vi "MainGUI.vi"() -> ()   [LabVIEW 2018]
uses:
  General/Controls/Queue Manager Actions.ctl
  General/Controls/MessagePacket.ctl
  General/Controls/QueueNames.ctl
  General/Controls/FGV Actions.ctl
  Hardware Mfg/Main Scan Processor Status.vi
  General/Controls/ScanType.ctl
  General/Controls/Set Get Controls.ctl
  Hardware Mfg/Thorlabs Translation Stages/Controls/Motion Translation Module Control.ctl
  Hardware Mfg/Axsun Laser/Axsun action.ctl
  Hardware Mfg/AlazarTech SDK/Controls/Alazar Engine Actions.ctl
  General/Controls/Optical Parameters.ctl
  General/Controls/Vibratome Parameters.ctl
  General/Controls/Scan Direction.ctl
  General/Controls/Imaging Parameters.ctl
panel:
  in  "Status":string
  in  "Quit":bool
  in  "Scan Type":T1
  in  "Acquire":bool
  in  "Control Panel":enum32{"Scan", "Config", "Manual Contorls"}(tab)
  in  "Imaging Parameter":T2={"Raster Scan Direction"=enum."Bi Directional", "Pixel Dwell Time [Clock Cycles]"=1, "Flyback Time [Clock Cycles]"=0, "XY Center [um]"={"X"=1.0, "Y"=1.0}, "Pixel Step Size [um]"=1.0, "XY Image Size"=enum."256 x 256", "Custom"=FALSE, "Custom Size"={"X"=1, "Y"=1}, "Line Averages"=1} {"Line Averages" min=1 max=30 step=1; "Flyback Time [Clock Cycles]" max=10 step=1; "Pixel Step Size [um]" min=0.0 max=10.0 step=0.01; "Custom Size"."Y" min=1 max=30 step=1; "Custom Size"."X" min=1 max=30 step=1; "XY Center [um]"."Y" min=1.0 max=30.0 step=1.0; "XY Center [um]"."X" min=1.0 max=30.0 step=1.0; "Pixel Dwell Time [Clock Cycles]" max=10 step=1}
  in  "Vibratome":T4={"Z Bottom [mm]"=0.0, "Pre Cut Dwell [s]"=0.0, "Blade Frequency [RPM]"=0, "Slice Speed [mm/s]"=0.0, "Post Cut Dwell [s]"=0.0, "Ramp Time [s]"=0.0, "Start X [mm]"=0.0, "Start Y [mm]"=0.0, "Slice Length [mm]"=0.0, "Slice Axis"=enum."X Axis", "Controller VISA Ref"="COM4"}
  in  "Optical Parameters":T5
  in  "Center Galvos":bool
  out "Label Name":string[][](array[string])
  out "Control Class ID":u32[](array[numeric])
  out "Image":T6(plugin-control)
  # "Image Settings"
  # "X"
  # "X"
  # "Vibratome Settings"
  # "Optical Settings"
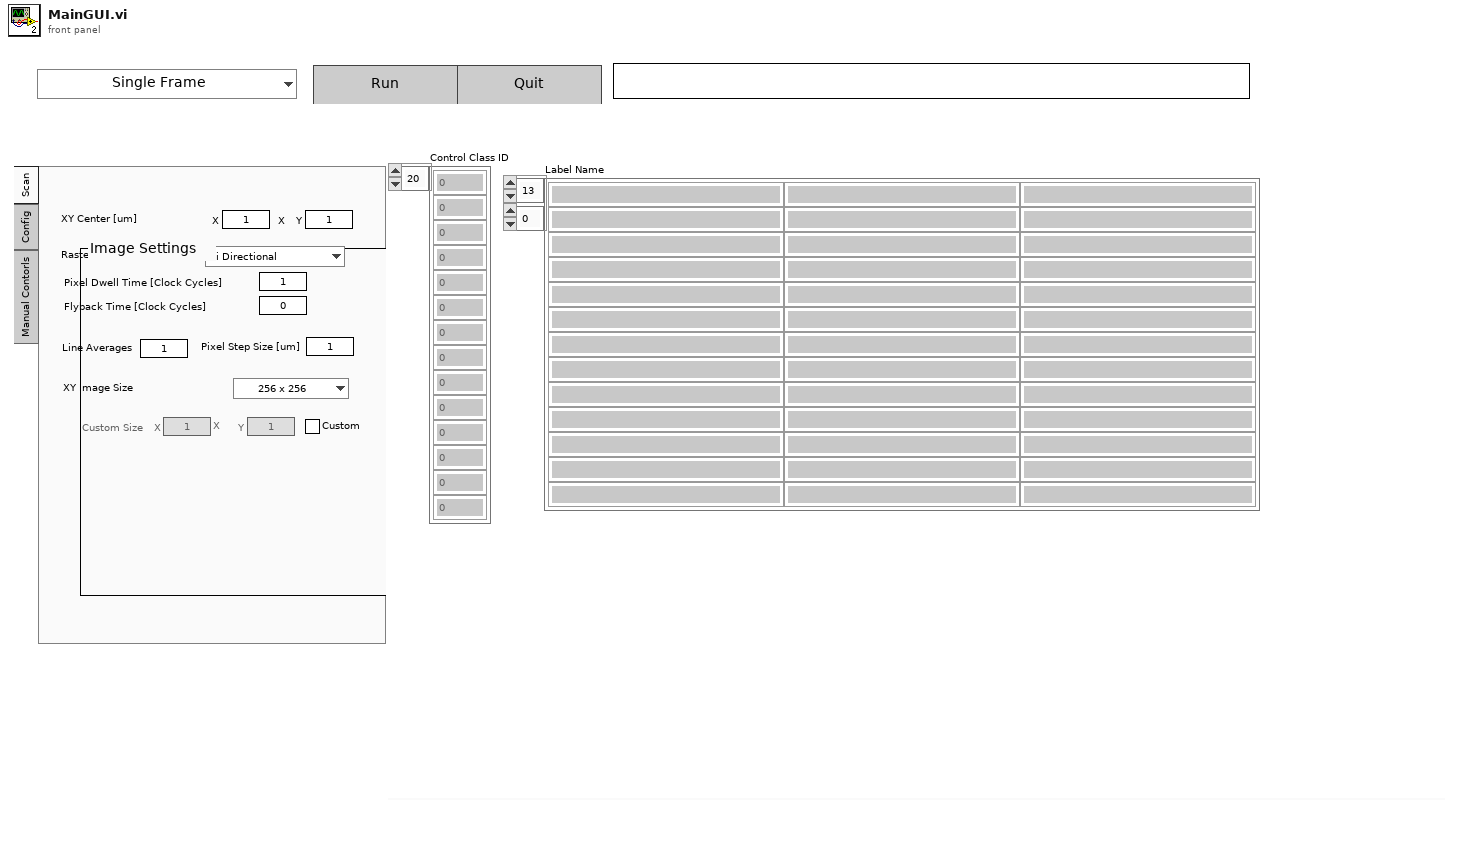
[diagram p1: front panel]
types:
  T1 = typedef "ScanType.ctl" = enum16{"Single Frame", "Continuous Frame", "ROI Line", "Vibratome", "Mosaic", "Mosaic + Slice"}
  T2 = typedef "Imaging Parameters.ctl" = cluster{"Raster Scan Direction":T3, "Pixel Dwell Time [Clock Cycles]":u16, "Flyback Time [Clock Cycles]":u16, "XY Center [um]":cluster{"X":dbl, "Y":dbl}, "Pixel Step Size [um]":dbl, "XY Image Size":enum16{"32 x 32", "64 x 64", "128 x 128", "256 x 256", "512 x 512", "1024 x 1024", "2048 x 2048"}, "Custom":bool, "Custom Size":cluster{"X":u16, "Y":u16}, "Line Averages":u8}
  T3 = typedef "Scan Direction.ctl" = enum16{"Uni Directional", "Bi Directional", "None"}
  T4 = typedef "Vibratome Parameters.ctl" = cluster{"Z Bottom [mm]":dbl, "Pre Cut Dwell [s]":dbl, "Blade Frequency [RPM]":u16, "Slice Speed [mm/s]":dbl, "Post Cut Dwell [s]":dbl, "Ramp Time [s]":dbl, "Start X [mm]":dbl, "Start Y [mm]":dbl, "Slice Length [mm]":dbl, "Slice Axis":enum16{"X Axis", "Y Axis", "Z Axis"}, "Controller VISA Ref":refnum<visa-resource-name>}
  T5 = typedef "Optical Parameters.ctl" = cluster{"Obj. Focal Length [mm]":dbl, "Scan Lens EFL[mm]":dbl, "Tube Lens EFL[mm]":dbl, "Galvo V Range (+/-)":dbl, "Galvo Max Half Angle [Deg]":dbl, "Max Galvo Range[%]":dbl}
  T6 = typedef "IMAQ Image.ctl" = refnum<image>
  T7 = typedef "QueueNames.ctl" = enum16{"Main GUI", "Main Scan Processor", "Main Display", "Main Table Stage GUI", "Main Table Stage Proc.", "Scan Engine", "Vibratome GUI", "Vibratome Processor", "Slice Engine"}
  T8 = typedef "Queue Manager Actions.ctl" = enum16{"Init", "Enqueue", "Enqueue All", "Preview Queue", "Dequeue", "Get Status", "Flush Queue", "Flush All Queues", "Release All Queues", "Release Queue", "Enqueue at Opposite End"}
  T9 = typedef "MessagePacket.ctl" = cluster{"Message":string, "Parameter":variant}
  T10 = typedef "FGV Actions.ctl" = enum16{"Init", "Set", "Get", "Clear"}
  T11 = typedef "System Parameters.ctl" = cluster{"Optical Parameters":T5, "Vibratome":T4, "Table Stages":T12, "Imaging Parameter":T2}
  T12 = typedef "Translation Stage Parameters.ctl" = cluster{"X Stage":T13, "Y Stage":T13, "Z Stage":T13}
  T13 = typedef "Translation Stage Cluster.ctl" = cluster{"Position":dbl, "Is.Enabled?":bool, "Is.Connected?":bool, "Device SN":string, "AccelerationMaximum":dbl, "VelocityMaximum":dbl, "Acceleration":dbl, "Velocity":dbl, "waitTimeout (ms)":i32, "Model":T14, "Is.Homed?":bool}
  T14 = typedef "Translation Stage Types.ctl" = enum16{"None", "Thorlabs LTS", "Thorlabs MLJ"}
  T15 = enum16{"32 x 32", "64 x 64", "128 x 128", "256 x 256", "512 x 512", "1024 x 1024", "2048 x 2048"}
  T16 = typedef "Axsun action.ctl" = enum16{"GetSystemStatus", "Clock delay", "GetLaserOnTime", "GetWaveLengthAtSweptTrigger", "Source current ON", "GetSerialNum", "GetControlVersion", "Laser ON", "Laser OFF", "Source current OFF", "Get laser handle", "Start Network Control Interface", "stop", "Create handle"}
  T17 = typedef "Alazar Engine Actions.ctl" = enum16{"Init", "Config Clock", "Config Ch", "Config Trig", "Config Non-FFT Acq.", "Non-FFT Acquire", "Load background from Non-FFT buffer", "enable background subtrac", "disable background subtrac", "load background from file", "load background from elsewhere", "start acquire", "background subtraction", "Config Acq.", "Acquire", "UnInit"}
  T18 = enum16{"Set Configuration", "Get Configuration", "Enable Motor", "Disable Motor", "Get Status", "Open Session", "Close Session", "Set Limits", "Get Limits"}
  T19 = enum16{"Configure channels", "Write Scan Pattern", "Start Galvo Task", "Is Task Done?", "Stop Galvo", "Uninit", "Init: Calc scan pattern"}
  T20 = typedef "Set Get Controls.ctl" = enum16{"Set", "Get"}
  T21 = typedef "Motion Translation Module Control.ctl" = enum16{"Init", "Home", "Status", "Velocity/Accel", "Position", "Jog", "Stop", "Uninit", "Enable", "Disable"}
  T22 = cluster{"X Stage":T13, "Y Stage":T13, "Z Stage":T13}
  T23 = typedef "Alazar parameters.ctl" = cluster{"Trigger Settings":cluster{"General Trigger Settings":T24, "Trigger Engine 1":T25, "Trigger Engine 2":T25}, "Capture Clock":T26, "Device ID":T27, "Ch A Input Control":T28, "Ch B Input Control":T28, "Acq Settings":T29, "Cluster":T30}
  T24 = typedef "General Trigger Settings.ctl" = cluster{"Trigger Operation":u32, "Coupling ID":u32, "Range ID":u32, "Delay":u32, "Timeout Ticks":u32, "Mode":u32, "Parameter":u32}
  T25 = typedef "Trigger Engine Controls.ctl" = cluster{"Trigger Engine":u32, "Source":u32, "Slope":u32, "Level":u32}
  T26 = typedef "Clock Controls.ctl" = cluster{"Sample Rate":u32, "Decimation":u32, "Source":u32, "Edge":u32}
  T27 = typedef "Alazar Device ID.ctl" = cluster{"System ID":u32, "Board ID":u32}
  T28 = typedef "Channel Input Controls.ctl" = cluster{"Channel":u8, "Coupling":u32, "Range":u32, "Impedance":u32}
  T29 = typedef "Alazar Acquisition Settings.ctl" = cluster{"Window Type":u32, "Record Length":u32, "Footer":u32, "Output Format":u32, "Offset":u32, "Records Per Buffer":u32, "Samples per record":u32, "Records Count (Records/Acq)":u32}
  T30 = typedef "Control cluster.ctl" = cluster{"FFT value magnification":dbl, "max queue size (-1, unlimited)":i32, "File Type":T31, "file path":path, "#A-lines to save":u32, "#Z pixels to save":u32, "ImageDescription":string, "Convert to U16?":bool}
  T31 = typedef "file type.ctl" = enum16{"text", "Tiff", "binary"}
  T32 = cluster{"General Trigger Settings":T24, "Trigger Engine 1":T25, "Trigger Engine 2":T25}
  T33 = typedef "Galvo parameters.ctl" = cluster{"Galvo HW Parameters":cluster{"Analog Out Channel":tag, "Min Voltage":dbl, "Max Voltage":dbl, "Pixel Clock Source":tag, "Sample Rate":dbl, "Line Clock Out Ch":tag}, "System Parameters":T11}
  T34 = cluster{"Analog Out Channel":tag, "Min Voltage":dbl, "Max Voltage":dbl, "Pixel Clock Source":tag, "Sample Rate":dbl, "Line Clock Out Ch":tag}
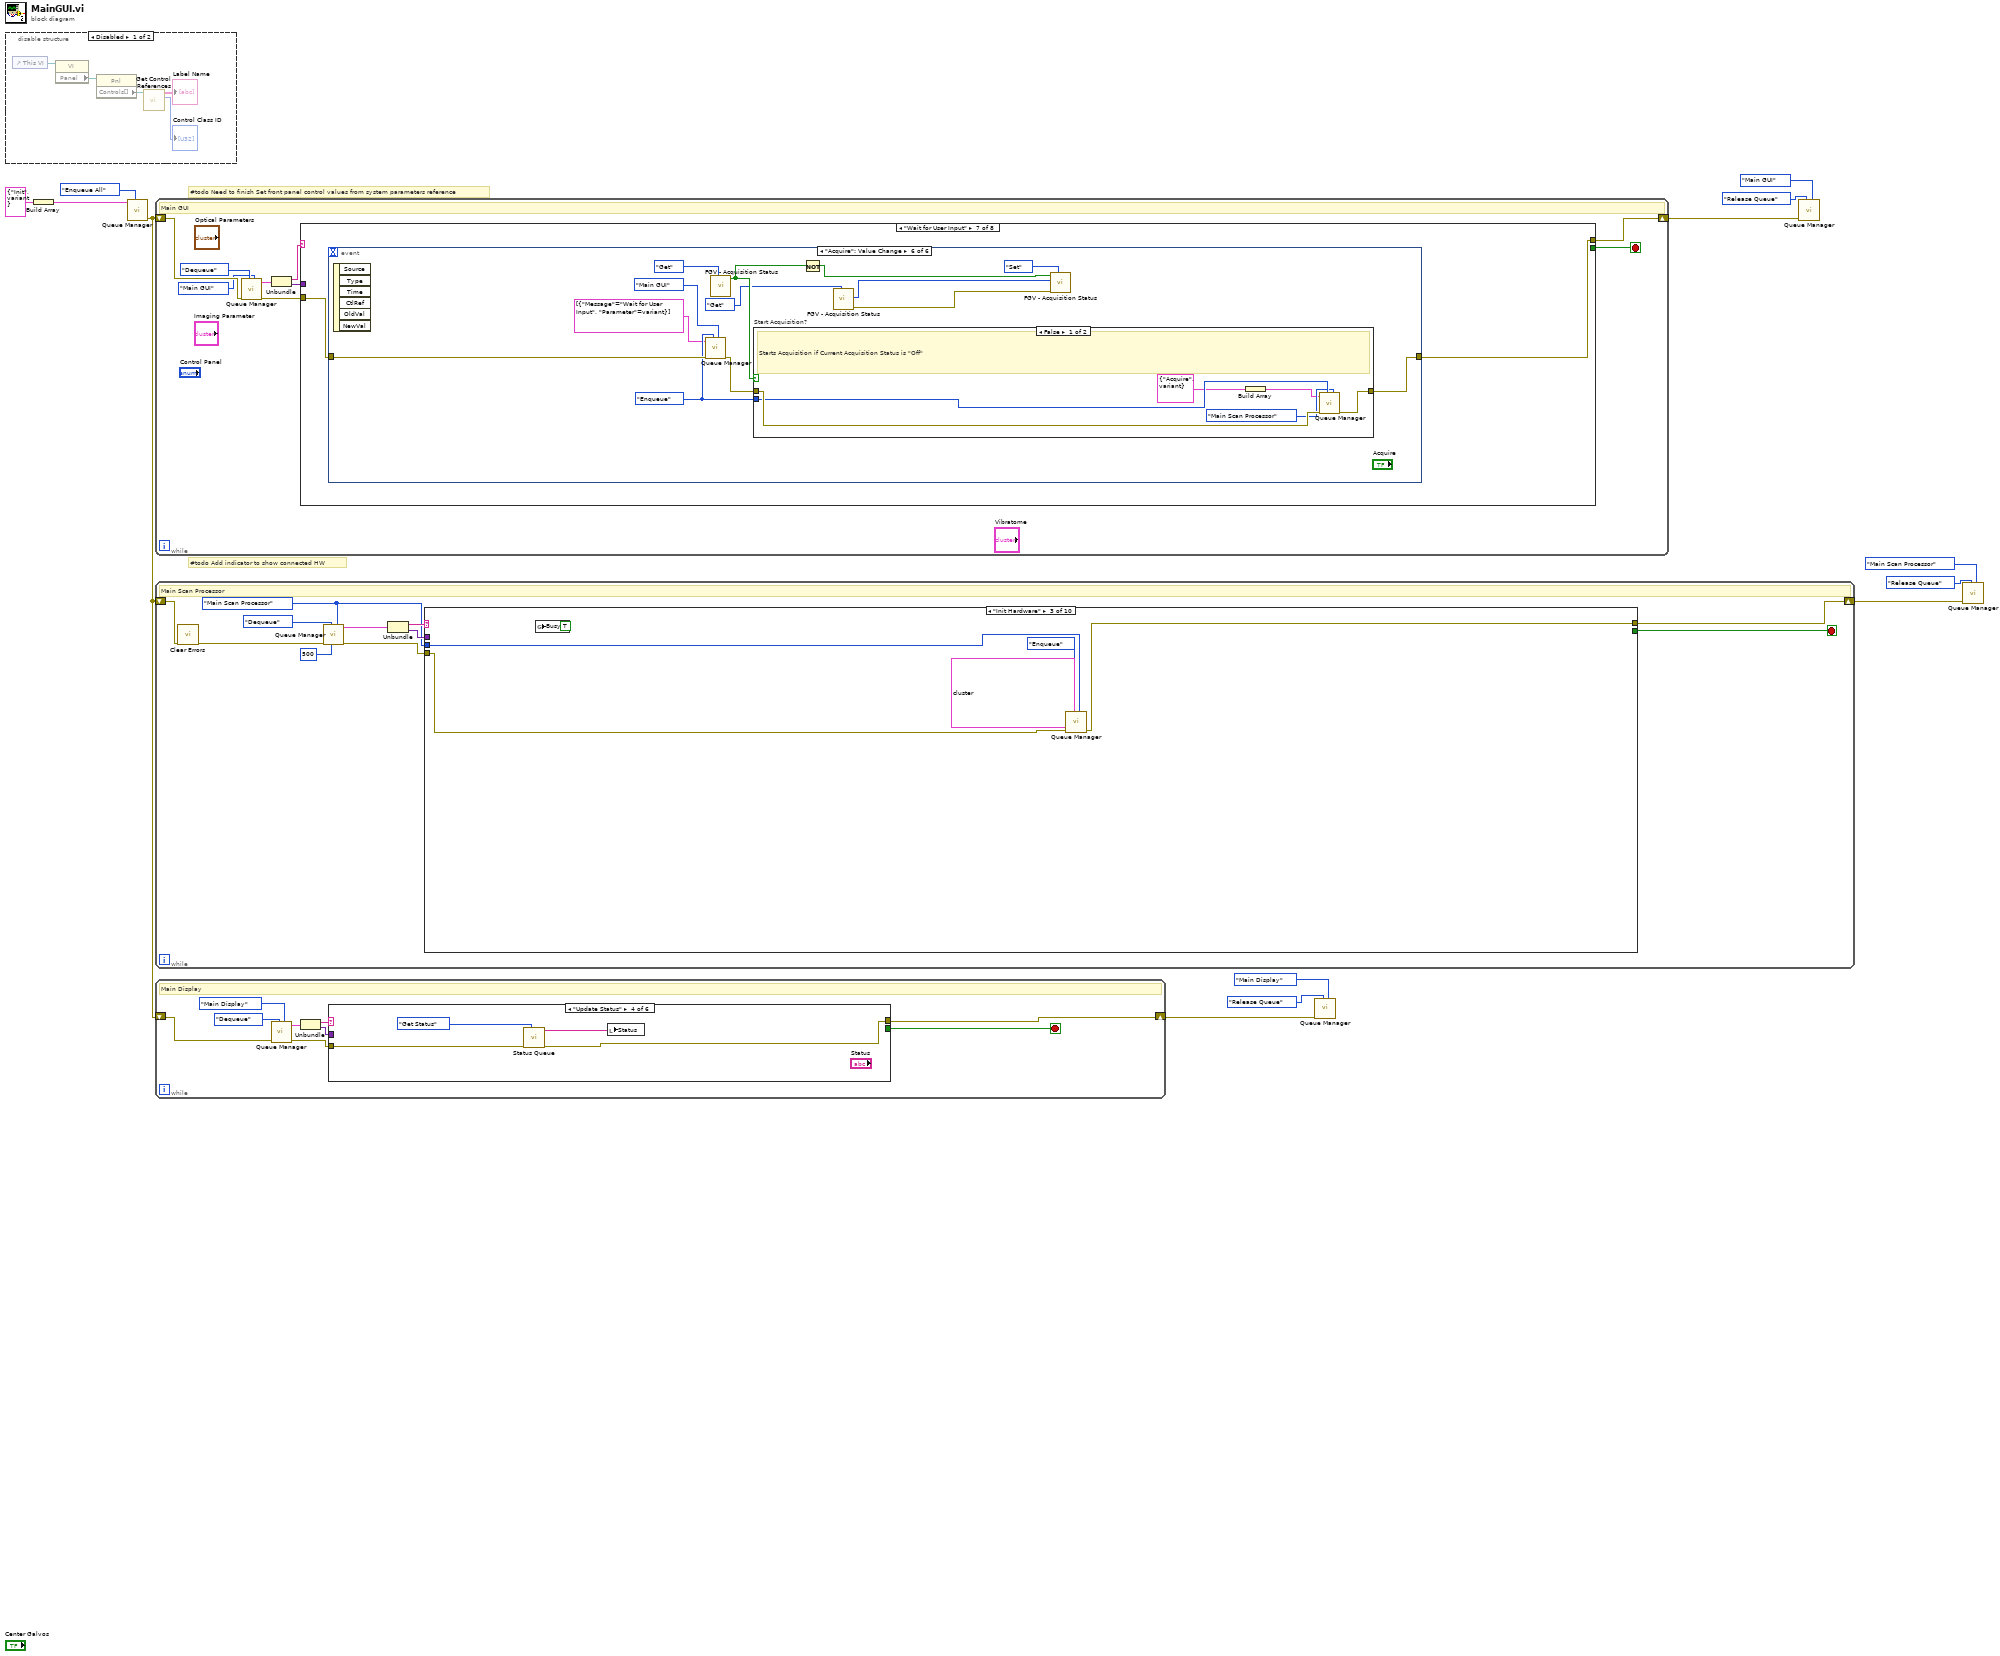
[diagram p0: block diagram]
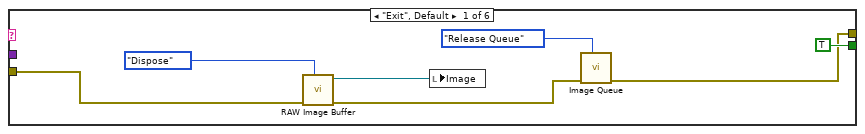
[diagram p3: hidden frame]
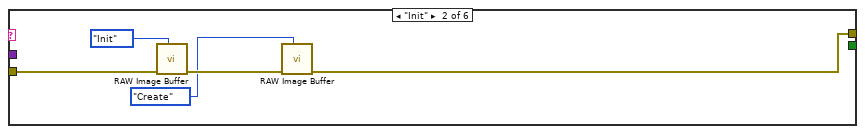
[diagram p4: hidden frame]
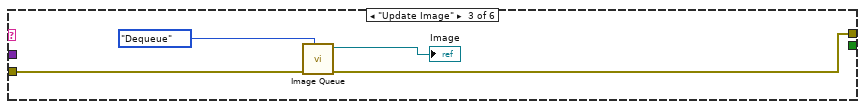
[diagram p5: hidden frame]
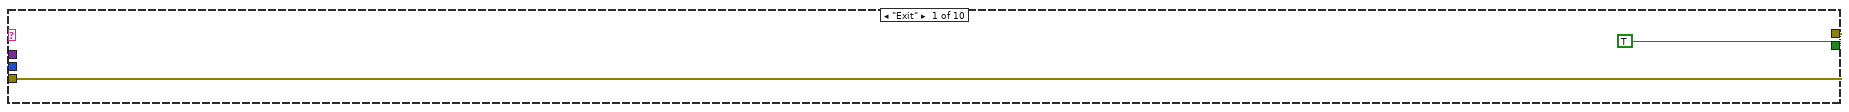
[diagram p8: hidden frame]
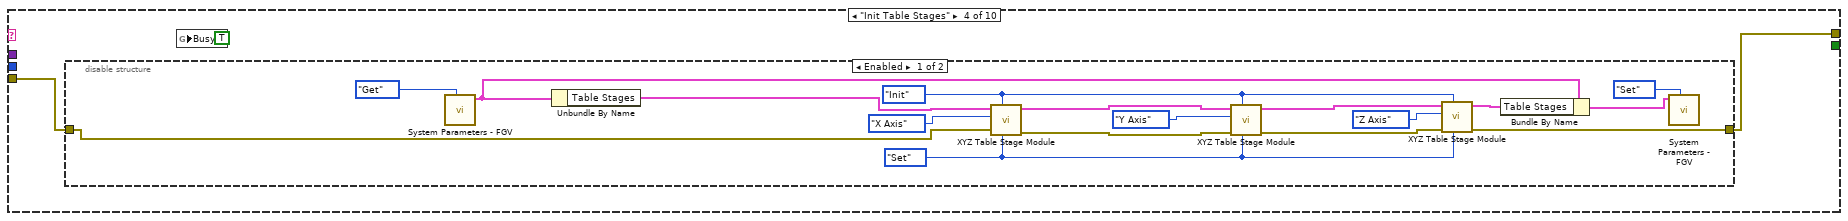
[diagram p10: hidden frame]
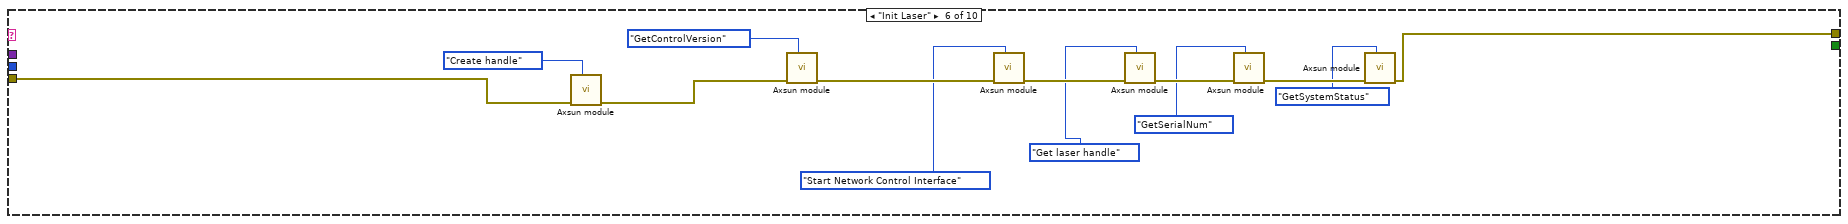
[diagram p13: hidden frame]
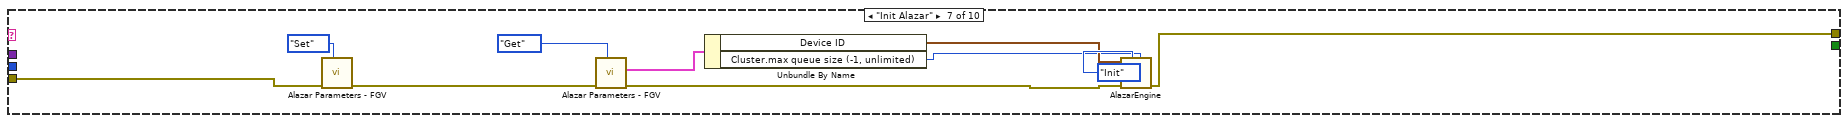
[diagram p14: hidden frame]
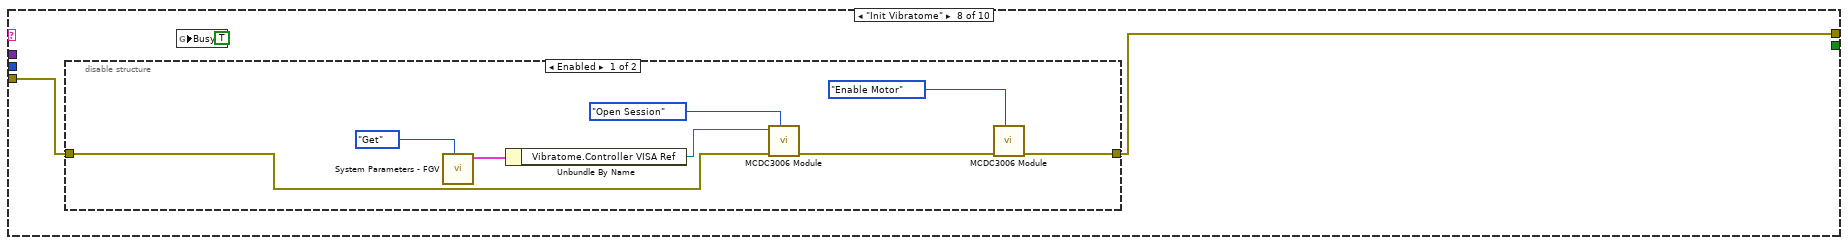
[diagram p15: hidden frame]
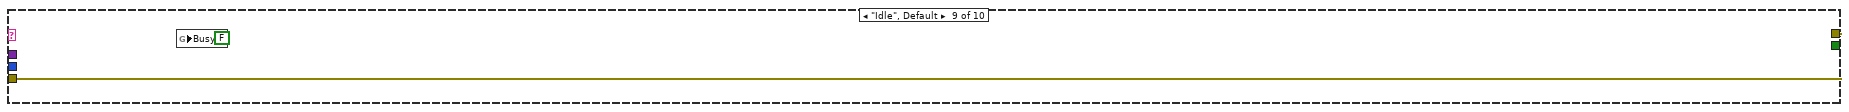
[diagram p17: hidden frame]
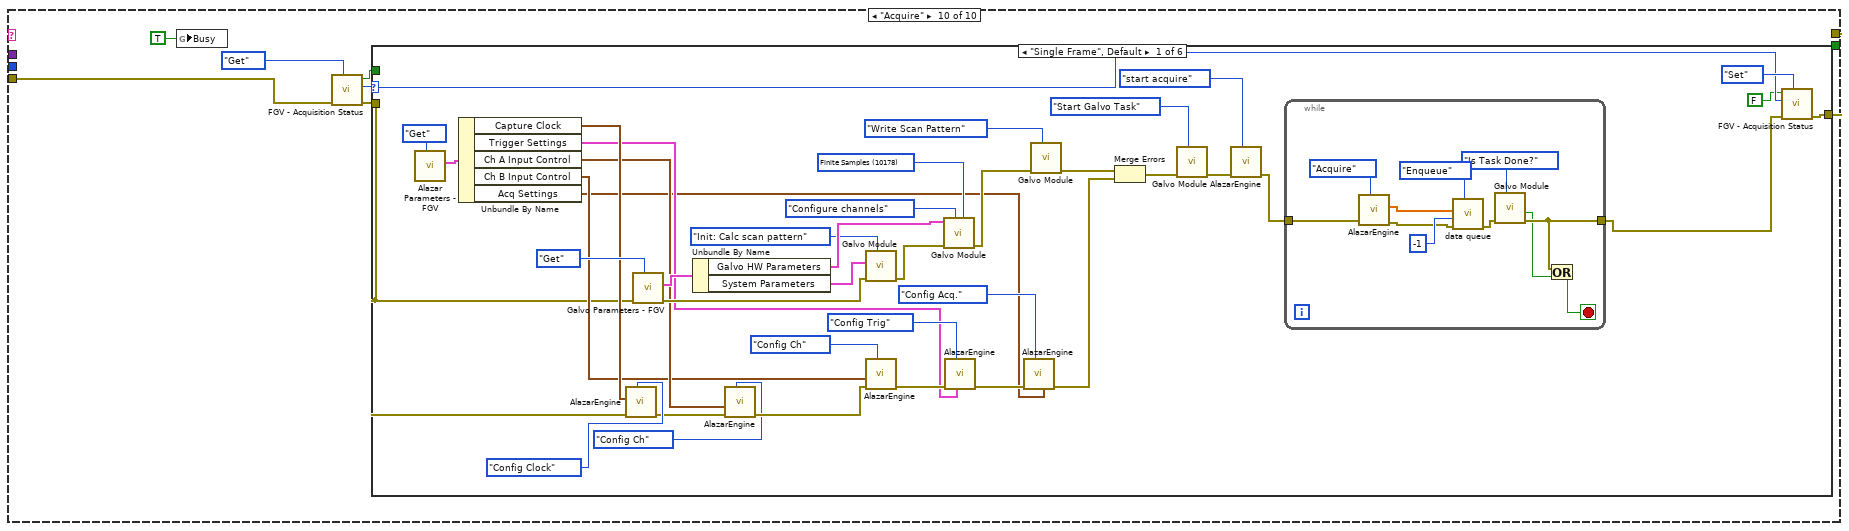
[diagram p18: hidden frame]
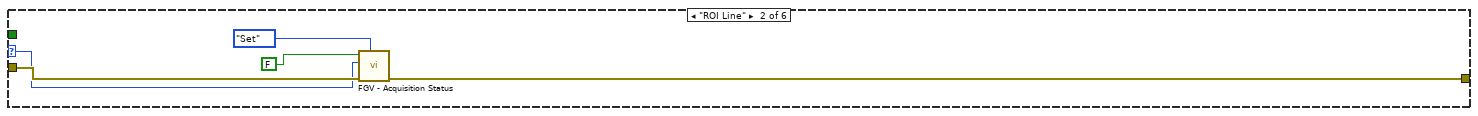
[diagram p19: hidden frame]
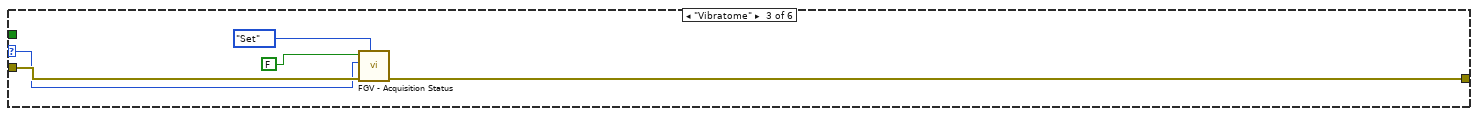
[diagram p20: hidden frame]
diagram:
  # "#todo Add indicator to show connected HW"
  # "#todo Need to finish Set front panel control values from system parameters reference"
  n1 = disable-structure shown="Disabled" {
    frame Disabled {
      n2 = control-ref of="This VI"() -> (w18:refnum<vi>)
      n3 = property class="VI"(reference=w18) -> ("Panel"=w17:refnum<vi>)  [unwired: 1 in, 2 out]
      n4 = property class="Pnl"(reference=w17) -> ("Controls[]"=w16:refnum<vi>[])  [unwired: 1 in, 2 out]
      n5 = call "Get Control References.vi"("Control References"=w16) -> ("Control Class ID"=→"Control Class ID":u32[], "Label Name"=→"Label Name":string[][])  [unwired: 8 in, 1 out]
    }
    frame Enabled {
    }
  }
  n6 = Build Array(T9 {"Message"="Init", "Parameter"=variant} ("Message Packet [In]")) -> (w11:T9[])
  n7 = call "Queue Manager.vi"("Action"=Queue_Manager_Actions."Enqueue All", "Message Packet Array"=w11) -> ("Error Out"=w1:errorcluster)  [unwired: 5 in, 4 out]
  n8 = while {
    shift-right: [w19] -> w10
    shift-left: w1 -> [w27]
    stop <- w22 stop-if-true
    # "Main GUI"
    n9 = call "Queue Manager.vi"("Queue Name"=QueueNames."Main GUI", "Action"=Queue_Manager_Actions."Dequeue", "Error In"=w27) -> ("Error Out"=w25:errorcluster, "Message Packet [Out]"=w24:T9)  [unwired: 4 in, 3 out]
    n10 = Unbundle(w24) -> ("Message"=w20:string, "Parameter"=w23:variant)
    n11 = case shown="\"Wait for User Input\"" w20 {
      tunnel: w25 -> [w32 w53 w58 w90 w97 w111 w123 w197]
      tunnel: w23 -> [_ _ _ _ _ _ _ _]
      tunnel: [w31 w49 w54 w86 w93 w109 w124 w198] -> w19
      tunnel: [_ _ _ _ _ _ _ TRUE] -> w22
      frame "Init" {
        n12 = call "Queue Manager.vi"("Queue Name"=QueueNames."Main GUI", "Action"=Queue_Manager_Actions."Enqueue", "Error In"=w32, "Message Packet Array"=T9[] [{"Message"="Init Variables", "Parameter"=variant}, {"Message"="Set Front Panel", "Parameter"=variant}, {"Message"="Update User Settings", "Parameter"=variant}, {"Message"="Configure Hardware", "Parameter"=variant}, {"Message"="Wait for Complete", "Parameter"=variant}, {"Message"="Wait for User Input", "Parameter"=variant}]) -> ("Error Out"=w31:errorcluster)  [unwired: 3 in, 4 out]
      }
      frame "Init Variables" {
        n13 = local write "Control Panel"(enum32{"Scan", "Config", "Manual Contorls"}."Scan" ("Control Panel")) -> ()
        n14 = call "Status Queue.vi"("Action"=Queue_Manager_Actions."Enqueue", "Error In"=w53, "Status Message [In]"="Initializing Variables...") -> ("Error Out"=w48:errorcluster)  [unwired: 7 in, 1 out]
        n15 = control-ref of="This VI"() -> (w51:refnum<vi>)
        n16 = call "Defer Panel Updates.vi"("Action"=enum16{"Init", "Freeze", "Unfreeze"}."Init", "Error In"=w48, "reference"=w51) -> ("Error Out"=w45:errorcluster)  [unwired: 8 in]
        n17 = call "System Parameters - FGV.vi"("Actions"=FGV_Actions."Init", "Error In"=w45) -> ("Error Out"=w41:errorcluster)  [unwired: 8 in, 1 out]
        n18 = call "Read Config from File.vi"("error in (no error)"=w41) -> ("error out"=w44:errorcluster, "System Parameters"=w42:T11)  [unwired: 9 in]
        n19 = control-ref of="Imaging Parameter"() -> (w34:refnum<vi>)
        n20 = call "System Parameters - FGV.vi"("Actions"=FGV_Actions."Set", "Error In"=w44, "System Parameters [In]"=w42) -> ("Error Out"=w37:errorcluster)  [unwired: 7 in, 1 out]
        n21 = call "Set Front Panel Custom Image Size Cluster Control.vi"("error in (no error)"=w37, "Enable/Disable"=FALSE, "Init"=TRUE, "Imaging Parameter"=w34) -> ("error IO"=w36:errorcluster)  [unwired: 7 in]
        n22 = call "FGV - Acquisition Status.vi"("Actions"=FGV_Actions."Init", "Error In"=w36) -> ("Error Out"=w49:errorcluster, "Scan Type [Out]"=w39:T1)  [unwired: 7 in, 1 out]
        n23 = local write "Scan Type"(w39) -> ()
      }
      frame "Set Front Panel" {
        n24 = call "Status Queue.vi"("Action"=Queue_Manager_Actions."Enqueue", "Error In"=w58, "Status Message [In]"="Setting Front Panel Controls...") -> ("Error Out"=w59:errorcluster)  [unwired: 7 in, 1 out]
        n25 = call "Defer Panel Updates.vi"("Action"=enum16{"Init", "Freeze", "Unfreeze"}."Freeze", "Error In"=w59) -> ("Error Out"=w67:errorcluster)  [unwired: 9 in]
        n26 = call "FGV - Acquisition Status.vi"("Actions"=FGV_Actions."Get", "Error In"=w67) -> ("Error Out"=w64:errorcluster, "Scan Type [Out]"=w62:T1, "Status Out"=w63:bool)  [unwired: 7 in]
        n27 = case "Acquiring?" shown="False" w63 {
          tunnel: [w71 w76] -> w65
          tunnel: w64 -> [w72 w76]
          tunnel: w62 -> [w70 _]
          frame False {
            # "Non-Acquiring FP States"
            n28 = disable-structure shown="Enabled" {
              disable-tunnel: w72 -> [w75 _]
              disable-tunnel: [w74 _] -> w71
              disable-tunnel: w70 -> [w73 _]
              frame Enabled {
                n29 = call "Set Main GUI for Different Acquire States.vi"("Error In"=w75, "Scan Type"=w73) -> ("Error Out"=w74:errorcluster)  [unwired: 9 in]
              }
              frame Disabled {
              }
            }
          }
          frame True {
            # "Acquiring FP States"
          }
        }
        n30 = call "Defer Panel Updates.vi"("Action"=enum16{"Init", "Freeze", "Unfreeze"}."Unfreeze", "Error In"=w65) -> ("Error Out"=w55:errorcluster)  [unwired: 9 in]
        n31 = call "Status Queue.vi"("Action"=Queue_Manager_Actions."Enqueue", "Error In"=w55, "Status Message [In]"="Finished Setting Front Panel.") -> ("Error Out"=w54:errorcluster)  [unwired: 7 in, 1 out]
      }
      frame "Update User Settings" {
        n32 = call "Status Queue.vi"("Action"=Queue_Manager_Actions."Enqueue", "Error In"=w90, "Status Message [In]"="Loading User Settings...") -> ("Error Out"=w88:errorcluster)  [unwired: 7 in, 1 out]
        n33 = call "Defer Panel Updates.vi"("Action"=enum16{"Init", "Freeze", "Unfreeze"}."Freeze", "Error In"=w88) -> ("Error Out"=w85:errorcluster)  [unwired: 9 in]
        n34 = call "System Parameters - FGV.vi"("Actions"=FGV_Actions."Get", "Error In"=w85) -> ("Error Out"=w79:errorcluster, "System Parameters"=w83:T11)  [unwired: 8 in]
        n35 = Unbundle By Name(w83) -> ("Optical Parameters"=w82:T5, "Vibratome"=w81:T4, "Imaging Parameter"=w80:T2)
        n36 = call "Set Front Panel Custom Image Size Cluster Control.vi"("error in (no error)"=w79, "Enable/Disable"=TRUE) -> ("error IO"=w78:errorcluster)  [unwired: 9 in]
        n37 = local write "Optical Parameters"(w82) -> ()
        n38 = local write "Vibratome"(w81) -> ()
        n39 = local write "Imaging Parameter"(w80) -> ()
        n40 = call "Defer Panel Updates.vi"("Action"=enum16{"Init", "Freeze", "Unfreeze"}."Unfreeze", "Error In"=w78) -> ("Error Out"=w86:errorcluster)  [unwired: 9 in]
      }
      frame "Configure Hardware" {
        n41 = call "Status Queue.vi"("Action"=Queue_Manager_Actions."Enqueue", "Error In"=w97, "Status Message [In]"="Initializing Hardware...") -> ("Error Out"=w96:errorcluster)  [unwired: 7 in, 1 out]
        n42 = Build Array(T9 {"Message"="Init Hardware", "Parameter"=variant} ("Message Packet [In]")) -> (w94:T9[])
        n43 = call "Queue Manager.vi"("Queue Name"=QueueNames."Main Scan Processor", "Action"=Queue_Manager_Actions."Enqueue", "Error In"=w96, "Message Packet Array"=w94) -> ("Error Out"=w93:errorcluster)  [unwired: 3 in, 4 out]
      }
      frame "Wait for Complete" {
        n44 = call "TickTock.vi"("Error In"=w111) -> ("Error Out"=w107:errorcluster, "Current Time (Out)"=w106:timestamp)  [unwired: 8 in, 1 out]
        n45 = while {
          shift-right: [w114] -> w108
          shift-left: w107 -> [w122]
          tunnel: w106 -> [w121]
          tunnel: [w112] -> w105
          stop <- w113 stop-if-true
          n46 = call "Inline Wait.vi"("Error In"=w122, "milliseconds to wait"=u32 100) -> ("Error Out"=w118:errorcluster)  [unwired: 9 in]
          n47 = call "TickTock.vi"("Error In"=w118, "Current Time (In)"=w121) -> ("Error Out"=w114:errorcluster, "dt"=w120:dbl)  [unwired: 7 in, 1 out]
          n48 = global read "Main Scan Processor Status.vi" "Busy"() -> (w116:bool)
          n49 = Greater?(x=60000.0, y=w120) -> (0:w112:bool)
          n50 = Not(x=w116) -> (.not. x?=w115:bool)
          n51 = Or(x=w112, y=w115) -> (x .or. y?=w113:bool)
        }
        n52 = Select(t="Completed." ("Status Message [In]"), s=w105, f="Operation timed out." ("Status Message [In]")) -> (s? t:f=w102:string)
        n53 = call "Status Queue.vi"("Action"=Queue_Manager_Actions."Enqueue", "Error In"=w108, "Status Message [In]"=w102) -> ("Error Out"=w109:errorcluster)  [unwired: 7 in, 1 out]
      }
      frame "Wait for User Input" {
        n54 = event shown="[5] \"Acquire\": Value Change" {
          selector: _ -> [_ _ _ _ _ _]
          dyn-events: _ -> [_ _ _ _ _ _]
          timeout: _ -> [_ _ _ _ _ _]
          tunnel: [w125 w135 w141 w157 w169 w184] -> w124
          tunnel: w123 -> [w125 w129 w143 w154 w173 w186]
          event Timeout {
            n55 = event-data() -> ()  [unwired: 1 in, 3 out]
          }
          event "Quit": Value Change {
            n56 = event-data() -> ()  [unwired: 1 in, 1 out]
            n57 = call "Status Queue.vi"("Action"=Queue_Manager_Actions."Enqueue", "Error In"=w129, "Status Message [In]"="Exiting Software...") -> ("Error Out"=w128:errorcluster)  [unwired: 7 in, 1 out]
            n58 = call "Set Main GUI for Different Acquire States.vi"("Error In"=w128, "Scan Type"=ScanType."Single Frame" ("Scan Type [Out]")) -> ("Error Out"=w127:errorcluster)  [unwired: 9 in]
            n59 = Build Array(T9 {"Message"="Exit", "Parameter"=variant} ("Message Packet [In]")) -> (w132:T9[])
            n60 = call "Queue Manager.vi"("Action"=Queue_Manager_Actions."Enqueue All", "Error In"=w127, "Message Packet Array"=w132) -> ("Error Out"=w135:errorcluster)  [unwired: 4 in, 4 out]
          }
          event "Image": Value Change {
            w144 = 2 items=["No Event"=0, "Click Event"=1, "Draw Event"=2, "Size Event"=4, "Scroll Event"=5, "Double Click Event"=8]
            n61 = event-data() -> ("CtlRef"=w136:refnum<vi>)  [unwired: 1 in, 5 out]
            n62 = Build Array(w144) -> (w145:i32[])
            n63 = invoke class="ImageControl" method="Get Last Event"(reference=w136, error in=w143, "Which Events"=w145) -> (error out=w142:errorcluster)  [unwired: 5 in, 7 out]
            n64 = Build Array(T9 {"Message"="Wait for User Input", "Parameter"=variant} ("Message Packet [In]")) -> (w137:T9[])
            n65 = call "Queue Manager.vi"("Queue Name"=QueueNames."Main GUI", "Action"=Queue_Manager_Actions."Enqueue", "Error In"=w142, "Message Packet Array"=w137) -> ("Error Out"=w141:errorcluster)  [unwired: 3 in, 4 out]
          }
          event Value Change {
            n66 = event-data() -> ("NewVal"=w149:T15)  [unwired: 1 in]
            n67 = Add(x=w149, y=5) -> (x+y=w163:i32)
            n68 = Power Of 2(x=w163) -> (2^x=w162:dbl)
            n69 = call "System Parameters - FGV.vi"("Actions"=FGV_Actions."Get", "Error In"=w154) -> ("Error Out"=w153:errorcluster, "System Parameters"=w151:T11)  [unwired: 8 in]
            n70 = Bundle By Name(cluster=w151, "Imaging Parameter.XY Image Size"=w149) -> (w150:T11)
            n71 = local read "Imaging Parameter"() -> (w148:T2)
            n72 = To Unsigned Word Integer(number=w162) -> (unsigned 16bit integer=w146:u16)
            n73 = Bundle By Name(cluster=w148, "Custom Size.X"=w146, "Custom Size.Y"=w146) -> (w147:T2)
            n74 = local write "Imaging Parameter"(w147) -> ()
            n75 = call "System Parameters - FGV.vi"("Actions"=FGV_Actions."Set", "Error In"=w153, "System Parameters [In]"=w150) -> ("Error Out"=w152:errorcluster)  [unwired: 7 in, 1 out]
            n76 = Build Array(T9 {"Message"="Wait for User Input", "Parameter"=variant} ("Message Packet [In]")) -> (w158:T9[])
            n77 = call "Queue Manager.vi"("Queue Name"=QueueNames."Main GUI", "Action"=Queue_Manager_Actions."Enqueue", "Error In"=w152, "Message Packet Array"=w158) -> ("Error Out"=w157:errorcluster)  [unwired: 3 in, 4 out]
          }
          event Value Change {
            n78 = event-data() -> ()  [unwired: 1 in, 6 out]
            n79 = call "FGV - Acquisition Status.vi"("Actions"=FGV_Actions."Get") -> ("Status Out"=w168:bool)  [unwired: 8 in, 2 out]
            n80 = call "FGV - Acquisition Status.vi"("Actions"=FGV_Actions."Set", "Scan Type [In]"="Scan Type", "Status In"=w168) -> ()  [unwired: 6 in, 3 out]
            n81 = call "Queue Manager.vi"("Queue Name"=QueueNames."Main GUI", "Action"=Queue_Manager_Actions."Enqueue", "Error In"=w173, "Message Packet Array"=T9[] [{"Message"="Set Front Panel", "Parameter"=variant}, {"Message"="Wait for User Input", "Parameter"=variant}]) -> ("Error Out"=w169:errorcluster)  [unwired: 3 in, 4 out]
          }
          event "Acquire": Value Change {
            w183 = Queue_Manager_Actions."Enqueue" ("Action")
            n82 = event-data() -> ()  [unwired: 1 in, 6 out]
            n83 = call "Queue Manager.vi"("Queue Name"=QueueNames."Main GUI", "Action"=w183, "Error In"=w186, "Message Packet Array"=T9[] [{"Message"="Wait for User Input", "Parameter"=variant}]) -> ("Error Out"=w185:errorcluster)  [unwired: 3 in, 4 out]
            n84 = call "FGV - Acquisition Status.vi"("Actions"=FGV_Actions."Get") -> ("Status Out"=w177:bool)  [unwired: 8 in, 2 out]
            n85 = case "Start Acquisition?" shown="False" w177 {
              tunnel: w185 -> [w192 w193]
              tunnel: [w191 w193] -> w184
              tunnel: w183 -> [w190 _]
              frame False {
                # "Starts Acquisition if Current Acquisition Status is \"Off\""
                n86 = Build Array(T9 {"Message"="Acquire", "Parameter"=variant} ("Message Packet [In]")) -> (w187:T9[])
                n87 = call "Queue Manager.vi"("Queue Name"=QueueNames."Main Scan Processor", "Action"=w190, "Error In"=w192, "Message Packet Array"=w187) -> ("Error Out"=w191:errorcluster)  [unwired: 3 in, 4 out]
              }
              frame True {
                # "Stops Acquisition if Current Status is On"
              }
            }
            n88 = Not(x=w177) -> (.not. x?=w178:bool)
            n89 = call "FGV - Acquisition Status.vi"("Actions"=FGV_Actions."Get") -> ("Error Out"=w176:errorcluster, "Scan Type [Out]"=w174:T1)  [unwired: 8 in, 1 out]
            n90 = call "FGV - Acquisition Status.vi"("Actions"=FGV_Actions."Set", "Error In"=w176, "Scan Type [In]"=w174, "Status In"=w178) -> ()  [unwired: 5 in, 3 out]
          }
        }
      }
      frame "Exit", Default {
        n91 = call "System Parameters - FGV.vi"("Actions"=FGV_Actions."Get", "Error In"=w197) -> ("Error Out"=w196:errorcluster, "System Parameters"=w194:T11)  [unwired: 8 in]
        n92 = call "Write Config to File.vi"("error in (no error)"=w196, "System Parameters"=w194) -> ("error out"=w198:errorcluster)  [unwired: 9 in]
      }
    }
  }
  n93 = while {
    shift-right: [w204] -> w5
    shift-left: w1 -> [w209]
    stop <- w203 stop-if-true
    w202 = QueueNames."Main Scan Processor" ("Queue Name")
    # "Main Scan Processor"
    n94 = call <vilib>:"Clear Errors.vi"("error in (no error)"=w209) -> ("error out"=w200:errorcluster)  [unwired: 5 in, 1 out]
    n95 = call "Queue Manager.vi"("Queue Name"=w202, "timeout in ms (-1)"=500, "Action"=Queue_Manager_Actions."Dequeue", "Error In"=w200) -> ("Error Out"=w208:errorcluster, "Message Packet [Out]"=w207:T9)  [unwired: 3 in, 3 out]
    n96 = Unbundle(w207) -> ("Message"=w206:string, "Parameter"=w205:variant)
    n97 = case shown="\"Init Hardware\"" w206 {
      tunnel: w208 -> [w211 w213 w219 w222 w241 w243 w262 w266 w278 w280]
      tunnel: w205 -> [_ _ _ _ _ _ _ _ _ _]
      tunnel: [w211 w213 w218 w221 w241 w242 w255 w265 w278 w285] -> w204
      tunnel: [TRUE _ _ _ _ _ _ _ _ _] -> w203
      tunnel: w202 -> [_ _ w217 _ _ _ _ _ _ _]
      frame "Exit" {
      }
      frame "Init" {
      }
      frame "Init Hardware" {
        n98 = global write "Main Scan Processor Status.vi" "Busy"(TRUE ("Busy")) -> ()
        n99 = call "Queue Manager.vi"("Queue Name"=w217, "Action"=Queue_Manager_Actions."Enqueue", "Error In"=w219, "Message Packet Array"=T9[] [{"Message"="Init Table Stages", "Parameter"=variant}, {"Message"="Init DAQ", "Parameter"=variant}, {"Message"="Init Vibratome", "Parameter"=variant}, {"Message"="Idle", "Parameter"=variant}, {"Message"="Init Laser", "Parameter"=variant}, {"Message"="Init Alazar", "Parameter"=variant}]) -> ("Error Out"=w218:errorcluster)  [unwired: 3 in, 4 out]
      }
      frame "Init Table Stages" {
        n100 = disable-structure shown="Enabled" {
          disable-tunnel: w222 -> [w230 w240]
          disable-tunnel: [w229 w240] -> w221
          frame Enabled {
            w231 = Set_Get_Controls."Set" ("Set/Get")
            w237 = Motion_Translation_Module_Control."Init" ("Action")
            n101 = call "System Parameters - FGV.vi"("Actions"=FGV_Actions."Get") -> ("System Parameters"=w225:T11)  [unwired: 9 in, 1 out]
            n102 = Unbundle By Name(w225) -> ("Table Stages"=w227:T12)
            n103 = call "XYZ Table Stage Module.vi"("Set/Get"=w231, "Action"=w237, "Error In"=w230, "Axis"=enum16{"X Axis", "Y Axis", "Z Axis"}."X Axis", "Table Stages"=w227) -> ("Error Out"=w239:errorcluster, "Table Stages Out"=w236:T22)  [unwired: 5 in]
            n104 = call "XYZ Table Stage Module.vi"("Set/Get"=w231, "Action"=w237, "Error In"=w239, "Axis"=enum16{"X Axis", "Y Axis", "Z Axis"}."Y Axis", "Table Stages"=w236) -> ("Error Out"=w238:errorcluster, "Table Stages Out"=w235:T22)  [unwired: 5 in]
            n105 = call "XYZ Table Stage Module.vi"("Set/Get"=w231, "Action"=w237, "Error In"=w238, "Axis"=enum16{"X Axis", "Y Axis", "Z Axis"}."Z Axis", "Table Stages"=w235) -> ("Error Out"=w229:errorcluster, "Table Stages Out"=w223:T22)  [unwired: 5 in]
            n106 = Bundle By Name(cluster=w225, "Table Stages"=w223) -> (w224:T11)
            n107 = call "System Parameters - FGV.vi"("Actions"=FGV_Actions."Set", "System Parameters [In]"=w224) -> ()  [unwired: 8 in, 2 out]
          }
          frame Disabled {
          }
        }
        n108 = global write "Main Scan Processor Status.vi" "Busy"(TRUE ("Busy")) -> ()
      }
      frame "Init DAQ" {
      }
      frame "Init Laser" {
        n109 = call "Axsun module.vi"("Action"=Axsun_action."Create handle", "error in (no error)"=w243) -> ("error out"=w253:errorcluster)  [unwired: 8 in, 1 out]
        n110 = call "Axsun module.vi"("Action"=Axsun_action."GetControlVersion", "error in (no error)"=w253) -> ("error out"=w252:errorcluster)  [unwired: 8 in, 1 out]
        n111 = call "Axsun module.vi"("Action"=Axsun_action."Start Network Control Interface", "error in (no error)"=w252) -> ("error out"=w251:errorcluster)  [unwired: 8 in, 1 out]
        n112 = call "Axsun module.vi"("Action"=Axsun_action."Get laser handle", "error in (no error)"=w251) -> ("error out"=w250:errorcluster)  [unwired: 8 in, 1 out]
        n113 = call "Axsun module.vi"("Action"=Axsun_action."GetSerialNum", "error in (no error)"=w250) -> ("error out"=w249:errorcluster)  [unwired: 8 in, 1 out]
        n114 = call "Axsun module.vi"("Action"=Axsun_action."GetSystemStatus", "error in (no error)"=w249) -> ("error out"=w242:errorcluster)  [unwired: 8 in, 1 out]
      }
      frame "Init Alazar" {
        n115 = call "Alazar Parameters - FGV.vi"("Actions"=FGV_Actions."Set", "Error In"=w262) -> ("Error Out"=w261:errorcluster)  [unwired: 8 in, 1 out]
        n116 = call "Alazar Parameters - FGV.vi"("Actions"=FGV_Actions."Get", "Error In"=w261) -> ("Error Out"=w256:errorcluster, "Alazar parameters out"=w259:T23)  [unwired: 8 in]
        n117 = Unbundle By Name(w259) -> ("Device ID"=w258:T27, "Cluster.max queue size (-1, unlimited)"=w257:i32)
        n118 = call "AlazarEngine.vi"("max queue size (-1, unlimited)"=w257, "Action"=Alazar_Engine_Actions."Init", "error in (no error)"=w256, "Device ID"=w258) -> ("error out"=w255:errorcluster)  [unwired: 6 in, 1 out]
      }
      frame "Init Vibratome" {
        n119 = disable-structure shown="Enabled" {
          disable-tunnel: w266 -> [w272 w276]
          disable-tunnel: [w271 w276] -> w265
          frame Enabled {
            n120 = call "System Parameters - FGV.vi"("Actions"=FGV_Actions."Get") -> ("System Parameters"=w269:T11)  [unwired: 9 in, 1 out]
            n121 = Unbundle By Name(w269) -> ("Vibratome.Controller VISA Ref"=w268:refnum<visa-resource-name>)
            n122 = call "MCDC3006 Module.vi"("Actions"=T18."Open Session", "Error In"=w272, "VISA resource name"=w268) -> ("Error Out"=w274:errorcluster)  [unwired: 4 in, 4 out]
            n123 = call "MCDC3006 Module.vi"("Actions"=T18."Enable Motor", "Error In"=w274) -> ("Error Out"=w271:errorcluster)  [unwired: 5 in, 4 out]
          }
          frame Disabled {
          }
        }
        n124 = global write "Main Scan Processor Status.vi" "Busy"(TRUE ("Busy")) -> ()
      }
      frame "Idle", Default {
        n125 = global write "Main Scan Processor Status.vi" "Busy"(FALSE ("Busy")) -> ()
      }
      frame "Acquire" {
        n126 = global write "Main Scan Processor Status.vi" "Busy"(TRUE ("Busy")) -> ()
        n127 = call "FGV - Acquisition Status.vi"("Actions"=FGV_Actions."Get", "Error In"=w280) -> ("Error Out"=w281:errorcluster, "Scan Type [Out]"=w283:T1, "Status Out"=w282:bool)  [unwired: 7 in]
        n128 = case shown="\"Single Frame\", Default" w283 {
          selector: w283 -> [w323 w338 w343 w348 w353 _]
          tunnel: w281 -> [w288 w339 w344 w349 w354 w364]
          tunnel: [w324 w340 w345 w350 w355 w363] -> w285
          tunnel: w282 -> [_ _ _ _ _ w358]
          frame "Single Frame", Default {
            w314 = 10178 items=["Finite Samples"=10178, "Continuous Samples"=10123, "Hardware Timed Single Point"=12522] ("sample mode")
            n129 = call "Alazar Parameters - FGV.vi"("Actions"=FGV_Actions."Get") -> ("Alazar parameters out"=w300:T23)  [unwired: 9 in, 1 out]
            n130 = Unbundle By Name(w300) -> ("Capture Clock"=w299:T26, "Trigger Settings"=w298:T32, "Ch A Input Control"=w297:T28, "Ch B Input Control"=w296:T28, "Acq Settings"=w295:T29)
            n131 = call "AlazarEngine.vi"("Action"=Alazar_Engine_Actions."Config Clock", "error in (no error)"=w288, "Capture Clock"=w299) -> ("error out"=w303:errorcluster)  [unwired: 7 in, 1 out]
            n132 = call "Galvo Parameters - FGV.vi"("Actions"=FGV_Actions."Get", "Error In"=w288) -> ("Error Out"=w321:errorcluster, "Galvo parameters out"=w316:T33)  [unwired: 8 in]
            n133 = Unbundle By Name(w316) -> ("Galvo HW Parameters"=w319:T34, "System Parameters"=w320:T11)
            n134 = call "AlazarEngine.vi"("Action"=Alazar_Engine_Actions."Config Ch", "error in (no error)"=w303, "Ch Input Control"=w297) -> ("error out"=w310:errorcluster)  [unwired: 7 in, 1 out]
            n135 = call "Galvo Module.vi"("Action"=T19."Init: Calc scan pattern", "error in (no error)"=w321, "System Parameters"=w320) -> ("error out"=w317:errorcluster)  [unwired: 7 in, 1 out]
            n136 = call "AlazarEngine.vi"("Action"=Alazar_Engine_Actions."Config Ch", "error in (no error)"=w310, "Ch Input Control"=w296) -> ("error out"=w307:errorcluster)  [unwired: 7 in, 1 out]
            n137 = call "Galvo Module.vi"("sample mode"=w314, "Action"=T19."Configure channels", "error in (no error)"=w317, "Galvo HW Parameters"=w319) -> ("error out"=w318:errorcluster)  [unwired: 6 in, 1 out]
            n138 = call "AlazarEngine.vi"("Trigger Settings"=w298, "Action"=Alazar_Engine_Actions."Config Trig", "error in (no error)"=w307) -> ("error out"=w304:errorcluster)  [unwired: 7 in, 1 out]
            n139 = call "AlazarEngine.vi"("Acq Settings"=w295, "Action"=Alazar_Engine_Actions."Config Acq.", "error in (no error)"=w304) -> ("error out"=w293:errorcluster)  [unwired: 7 in, 1 out]
            n140 = call "Galvo Module.vi"("Action"=T19."Write Scan Pattern", "error in (no error)"=w318) -> ("error out"=w294:errorcluster)  [unwired: 8 in, 1 out]
            n141 = Merge Errors(w294, w293) -> (w290:errorcluster)
            n142 = call "Galvo Module.vi"("Action"=T19."Start Galvo Task", "error in (no error)"=w290) -> ("error out"=w289:errorcluster)  [unwired: 8 in, 1 out]
            n143 = call "AlazarEngine.vi"("Action"=Alazar_Engine_Actions."start acquire", "error in (no error)"=w289) -> ("error out"=w287:errorcluster)  [unwired: 8 in, 1 out]
            n144 = while {
              tunnel: w287 -> [w335]
              tunnel: [w328] -> w286
              stop <- w326 stop-if-true
              n145 = call "AlazarEngine.vi"("Action"=Alazar_Engine_Actions."Acquire", "error in (no error)"=w335) -> ("error out"=w331:errorcluster, "Buffer"=w329:sgl[])  [unwired: 8 in]
              n146 = call "data queue.vi"("Action"=Queue_Manager_Actions."Enqueue", "error in (no error)"=w331, "timeout in ms (-1)"=-1, "data in"=w329) -> ("error out"=w330:errorcluster)  [unwired: 4 in, 3 out]
              n147 = call "Galvo Module.vi"("Action"=T19."Is Task Done?", "error in (no error)"=w330) -> ("error out"=w328:errorcluster, "task done?"=w327:bool)  [unwired: 8 in]
              n148 = Or(x=w328, y=w327) -> (x .or. y?=w326:bool)
            }
            n149 = call "FGV - Acquisition Status.vi"("Actions"=FGV_Actions."Set", "Error In"=w286, "Scan Type [In]"=w323, "Status In"=FALSE) -> ("Error Out"=w324:errorcluster)  [unwired: 5 in, 2 out]
          }
          frame "ROI Line" {
            n150 = call "FGV - Acquisition Status.vi"("Actions"=FGV_Actions."Set", "Error In"=w339, "Scan Type [In]"=w338, "Status In"=FALSE) -> ("Error Out"=w340:errorcluster)  [unwired: 5 in, 2 out]
          }
          frame "Vibratome" {
            n151 = call "FGV - Acquisition Status.vi"("Actions"=FGV_Actions."Set", "Error In"=w344, "Scan Type [In]"=w343, "Status In"=FALSE) -> ("Error Out"=w345:errorcluster)  [unwired: 5 in, 2 out]
          }
          frame "Mosaic" {
            n152 = call "FGV - Acquisition Status.vi"("Actions"=FGV_Actions."Set", "Error In"=w349, "Scan Type [In]"=w348, "Status In"=FALSE) -> ("Error Out"=w350:errorcluster)  [unwired: 5 in, 2 out]
          }
          frame "Mosaic + Slice" {
            n153 = call "FGV - Acquisition Status.vi"("Actions"=FGV_Actions."Set", "Error In"=w354, "Scan Type [In]"=w353, "Status In"=FALSE) -> ("Error Out"=w355:errorcluster)  [unwired: 5 in, 2 out]
          }
          frame "Continuous Frame" {
            n154 = case "Load Test Image" shown="True" TRUE {
              tunnel: w364 -> [w372 w375]
              tunnel: [w372 w374] -> w361
              tunnel: [_ w373] -> w359
              frame False {
              }
              frame True {
                n155 = call "Load Test Image.vi"("Error In"=w375) -> ("Error Out"=w374:errorcluster, "Image"=w373:T6)  [unwired: 9 in]
              }
            }
            n156 = call "Image Queue.vi"("Action"=Queue_Manager_Actions."Enqueue", "Error In"=w361, "Image In"=w359) -> ("Error Out"=w357:errorcluster)  [unwired: 7 in, 1 out]
            n157 = case shown="True" w358 {
              tunnel: [w365 w371] -> w363
              tunnel: w357 -> [w365 w366]
              frame False {
              }
              frame True {
                n158 = Build Array(T9 {"Message"="Acquire", "Parameter"=variant} ("Message Packet [In]")) -> (w367:T9[])
                n159 = call "Queue Manager.vi"("Queue Name"=QueueNames."Main Scan Processor", "Action"=Queue_Manager_Actions."Enqueue", "Error In"=w366, "Message Packet Array"=w367) -> ("Error Out"=w371:errorcluster)  [unwired: 3 in, 4 out]
              }
            }
          }
        }
      }
    }
  }
  n160 = while {
    shift-right: [w377] -> w3
    shift-left: w1 -> [w382]
    stop <- w376 stop-if-true
    # "Main Display"
    n161 = call "Queue Manager.vi"("Queue Name"=QueueNames."Main Display", "Action"=Queue_Manager_Actions."Dequeue", "Error In"=w382) -> ("Error Out"=w381:errorcluster, "Message Packet [Out]"=w380:T9)  [unwired: 4 in, 3 out]
    n162 = Unbundle(w380) -> ("Message"=w379:string, "Parameter"=w378:variant)
    n163 = case shown="\"Update Status\"" w379 {
      tunnel: w381 -> [w389 w396 w400 w404 w405 w406]
      tunnel: w378 -> [_ _ _ _ _ _]
      tunnel: [w387 w392 w399 w403 w405 w406] -> w377
      tunnel: [TRUE _ _ _ _ _] -> w376
      frame "Exit", Default {
        n164 = call "RAW Image Buffer.vi"("Actions"=enum16{"Init", "Create", "Get", "Dispose"}."Dispose", "Error In"=w389) -> ("Error Out"=w388:errorcluster, "Image Out"=w385:T6)  [unwired: 8 in]
        n165 = local write "Image"(w385) -> ()
        n166 = call "Image Queue.vi"("Action"=Queue_Manager_Actions."Release Queue", "Error In"=w388) -> ("Error Out"=w387:errorcluster)  [unwired: 8 in, 1 out]
      }
      frame "Init" {
        n167 = call "RAW Image Buffer.vi"("Actions"=enum16{"Init", "Create", "Get", "Dispose"}."Init", "Error In"=w396) -> ("Error Out"=w395:errorcluster)  [unwired: 8 in, 1 out]
        n168 = call "RAW Image Buffer.vi"("Actions"=enum16{"Init", "Create", "Get", "Dispose"}."Create", "Error In"=w395) -> ("Error Out"=w392:errorcluster)  [unwired: 8 in, 1 out]
      }
      frame "Update Image" {
        n169 = call "Image Queue.vi"("Action"=Queue_Manager_Actions."Dequeue", "Error In"=w400) -> ("Error Out"=w399:errorcluster, "Image Out"=→"Image":T6)  [unwired: 8 in]
      }
      frame "Update Status" {
        n170 = call "Status Queue.vi"("Action"=Queue_Manager_Actions."Get Status", "Error In"=w404) -> ("Error Out"=w403:errorcluster, "Status Message [Out]"=w401:string)  [unwired: 8 in]
        n171 = local write "Status"(w401) -> ()
      }
      frame "Update Line Profile" {
      }
      frame "Idle" {
      }
    }
  }
  n172 = call "Queue Manager.vi"("Queue Name"=QueueNames."Main Display", "Action"=Queue_Manager_Actions."Release Queue", "Error In"=w3) -> ()  [unwired: 4 in, 5 out]
  n173 = call "Queue Manager.vi"("Queue Name"=QueueNames."Main GUI", "Action"=Queue_Manager_Actions."Release Queue", "Error In"=w10) -> ()  [unwired: 4 in, 5 out]
  n174 = call "Queue Manager.vi"("Queue Name"=QueueNames."Main Scan Processor", "Action"=Queue_Manager_Actions."Release Queue", "Error In"=w5) -> ()  [unwired: 4 in, 5 out]
